vi "Write NChan 1Sample 1D SGL.vi"(8 "error in (no error)":errorcluster, 10 "data":dbl[](array[numeric]), 11 "Analog Output in":refnum<class "Analog output.lvclass">) -> (0 "error out":errorcluster, 3 "Analog Output out":refnum<class "Analog output.lvclass">)   [LabVIEW 2009, in "MicroDAQ.lvlib" / "Analog output.lvclass"]
doc: "Writes const values to all channels."
uses:
  <instrlib>/MicroDAQ/Channel/Analog Output/Analog output.lvclass
  <instrlib>/MicroDAQ/Channel/Analog Output/Analog output.lvclass/Analog output.ctl
  <instrlib>/MicroDAQ/Channel/Channel.lvclass
  <instrlib>/MicroDAQ/Mlink library wraper/mlink.lvlib
  <instrlib>/MicroDAQ/MicroDAQ.lvlib
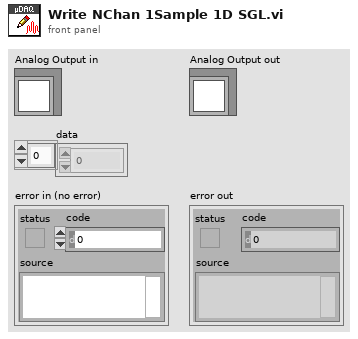
[diagram p1: front panel]
types:
  T1 = typedef "MicroDAQ.lvlib/Analo Range Enum.ctl" = enum16{"±10V", "0-10V", "±5V", "0-5V", "±5.12V", "±2.56V", "±2.5V", "±2V", "±1.24V", "±0.64V"}
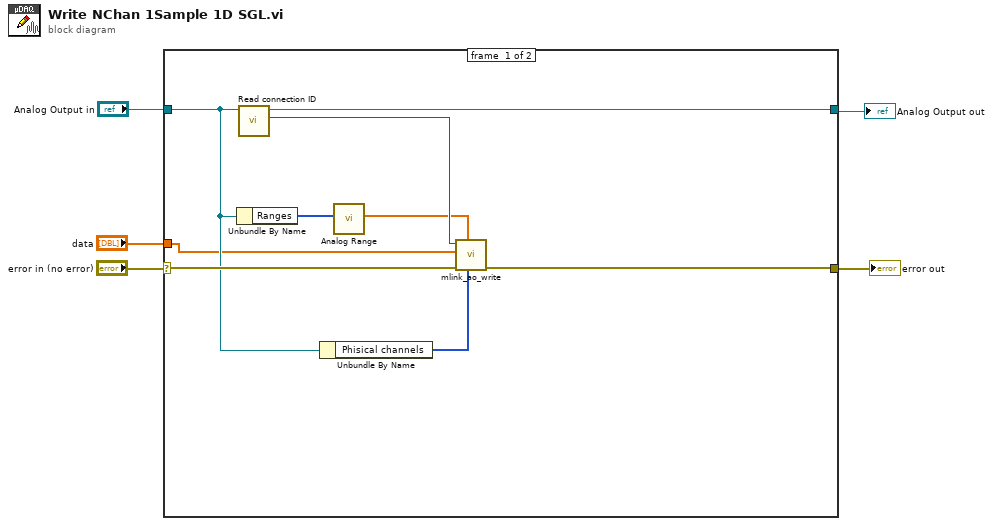
[diagram p0: block diagram]
diagram:
  n1 = case shown="No Error" "error in (no error)" {
    selector: "error in (no error)" -> [w12 w16]
    tunnel: [w8 w16] -> w4
    tunnel: [w14 w15] -> w1
    tunnel: "Analog Output in" -> [w11 w15]
    tunnel: "data" -> [w9 _]
    frame #0 {
      n2 = Unbundle By Name(w11) -> ("Ranges"=w7:T1[])
      n3 = call <instrlib>:"Read connection ID.vi"("Task in"=w11) -> ("connection ID"=w13:i32, "Task out"=w14:refnum<class "Analog output.lvclass">)  [unwired: 9 in]
      n4 = Unbundle By Name(w11) -> ("Phisical channels"=w10:u8[])
      n5 = call <instrlib>:"Analog Range.vi"("ranges in"=w7) -> ("range Array out"=w6:dbl[])  [unwired: 10 in]
      n6 = call <instrlib>:"mlink_ao_write.vi"("channels"=w10, "range"=w6, "error in (no error)"=w12, "data"=w9, "connection ID"=w13) -> ("error out"=w8:errorcluster)  [unwired: 5 in, 1 out]
    }
    frame #1 {
    }
  }
  "error out" <- w4
  "Analog Output out" <- w1
